vi "SATSPLNdll.vi"(8 "error in (no error)":errorcluster, 11 "z":dbl[](array[numeric])) -> (0 "error out":errorcluster, 1 "ln out":i32, 2 "herr out":string, 3 "ierr out":i32)   [LabVIEW 2015]
doc: "subroutine SATSPLNdll(z, ierr, herr, herr_length)\n\nCalculates the phase boundary of a mixture at a given composition,\nand the critical point, cricondentherm, and cricondenbar.\n\nINPUTS:\nz -- composition [array of mol frac]\n\nOUTPUTS:\nierr -- Error flag: 0 = Successful \nherr -- Error string (character*255)\nherr_length -- length of variable herr (default: 255)"
uses:
  REFPROP.dll
panel:
  # "REFPROP-SATSPLNdll.vi"
  # "void  SATSPLNdll(double *z, int32_t *ierr, CStr herr, int32_t *herr_length)"
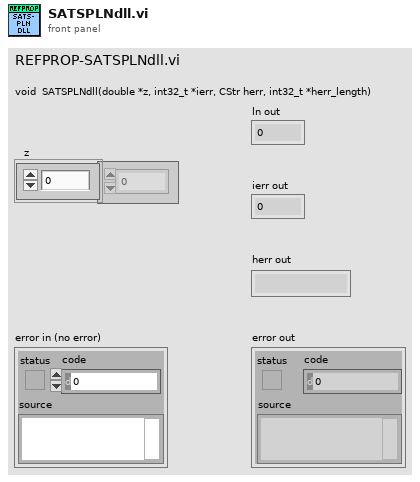
[diagram p1: front panel]
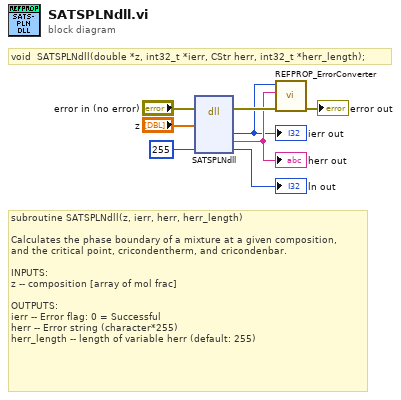
[diagram p0: block diagram]
diagram:
  # "void  SATSPLNdll(double *z, int32_t *ierr, CStr herr, int32_t *herr_length);"
  # "subroutine SATSPLNdll(z, ierr, herr, herr_length)\n\nCalculates the phase boundary of a mixture at a given composition,\nand the critical point, cricondentherm, and cricondenbar.\n\nINPUTS:\nz -- composition [array of mol frac]\n\nOUTPUTS:\nierr -- Error flag: 0 = Successful \nherr -- Error string (character*255)\nherr_length -- length of variable herr (default: 255)"
  n1 = dll-call lib="C:/Users/lauria/Desktop/REFPROP 10 LabVIEW Wrapper BETA/REFPROP/REFPROP.*" fn="SATSPLNdll"(error in="error in (no error)", "z"="z", "herr_length"=255 ("ln")) -> (error out=w5:errorcluster, "ierr"=w1:i32, "herr"=w2:string, "herr_length"=→"ln out":i32)  [unwired: 6 in, 1 out]
  "ierr out" <- w1
  "herr out" <- w2
  n2 = call "REFPROP_ErrorConverter.vi"("error in (no error)"=w5, "Error Message"=w2, "Error Code"=w1) -> ("error out"=→"error out":errorcluster)  [unwired: 8 in]
